vi "Kurven anzeigen.vi"() -> ()   [LabVIEW 2020, in "Grafik.lvlib"]
uses:
  Grafik.lvlib
  Visualisierungs Elemente/Button.ctl
  FT-IR/FGV FT-IR Gasliste Aktionen.ctl
  Messdaten/Aktionen FGV Messdaten.ctl
  Gaszuordnung AO/FGV Gaszuordnung Gas-Auswahl Aktion.ctl
  Messdaten/Messdaten.lvlib
  FT-IR/FT-IR.lvlib
  Gaszuordnung AO/Gaszuordnung AO.lvlib
  Allgemein/allgemeine Sub-VIs.lvlib
panel:
  in  "Clear":T1 caption="Beenden"
  in  "Beenden":T1
  in  "Komponenten":T2 {"Komponente 6" items=["---", "NO (3000) LP 191C", "NO2 (150) LP 191C (1of2)", "NO2 (2000) LP 191C (2of2)", "N2O (300) LP 191C (1of2)", "NH3 (300) LP 191C (1of2)", "NH3 (900,3000) LP 191C (2of2)", "HNCO (400) 191C", "H2O% (30) LP 191C", "Formaldehyde (70,500) LP 191C", "CO2 low% (4) LP 191C (2of2)", "CO2% (20) LP 191C (1of2)", "CO (700) LP 191C (1of3)", "CO% (1) LP 191C (2of3)", "Propylene (1000) LP 191C", "Aromatic HC C7 (500) LP 191C", "Ethylene (1000) LP 191C", "CH4 (250) LP 191C (1of2)", "CH4 (5000) LP 191C (2of2)", "Ethane (1000) LP 191C", "Acetylene (1000) LP 191C", "HNO2 (20) 191C", "MeOH (1000) 191C", "CO% (10) LP 191C (3of3)", "Formic Acid (100) 191C", "SO2 (500) LP 191C", "Acetaldehyde (1000) LP 191C", "COS (100) LP 191C", "1,3 butadiene (100) LP 191C", "Oil as Octane (200) LP 191C", "N2O (1000) LP 191C (2of2)", "Propane (200) LP 191C", "NO2 autorange (2000)", "CO autorange (100000)", "CH4 autorange (5000)", "NH3 autorange (3000)", "NOx autorange (3000)", "HCD (10000)", "NMHCD (10000)", "CO2% autorange (20)", "H2Oppm (300000)", "N2O autorange (1000)", "NMNEHCD (3000)", "Temp. Messzelle", "Druck Messzelle", "sBeam@2500", "Temp. HL zu FT-IR", "Temp. HL Extern SP1", "Austrittstemp. FT-IR", "Temp. Schaltschrank", "Konstant 0", "Konstant 50", "Konstant 100", "AK DUMMY"]; "Komponente 5" items=["---", "NO (3000) LP 191C", "NO2 (150) LP 191C (1of2)", "NO2 (2000) LP 191C (2of2)", "N2O (300) LP 191C (1of2)", "NH3 (300) LP 191C (1of2)", "NH3 (900,3000) LP 191C (2of2)", "HNCO (400) 191C", "H2O% (30) LP 191C", "Formaldehyde (70,500) LP 191C", "CO2 low% (4) LP 191C (2of2)", "CO2% (20) LP 191C (1of2)", "CO (700) LP 191C (1of3)", "CO% (1) LP 191C (2of3)", "Propylene (1000) LP 191C", "Aromatic HC C7 (500) LP 191C", "Ethylene (1000) LP 191C", "CH4 (250) LP 191C (1of2)", "CH4 (5000) LP 191C (2of2)", "Ethane (1000) LP 191C", "Acetylene (1000) LP 191C", "HNO2 (20) 191C", "MeOH (1000) 191C", "CO% (10) LP 191C (3of3)", "Formic Acid (100) 191C", "SO2 (500) LP 191C", "Acetaldehyde (1000) LP 191C", "COS (100) LP 191C", "1,3 butadiene (100) LP 191C", "Oil as Octane (200) LP 191C", "N2O (1000) LP 191C (2of2)", "Propane (200) LP 191C", "NO2 autorange (2000)", "CO autorange (100000)", "CH4 autorange (5000)", "NH3 autorange (3000)", "NOx autorange (3000)", "HCD (10000)", "NMHCD (10000)", "CO2% autorange (20)", "H2Oppm (300000)", "N2O autorange (1000)", "NMNEHCD (3000)", "Temp. Messzelle", "Druck Messzelle", "sBeam@2500", "Temp. HL zu FT-IR", "Temp. HL Extern SP1", "Austrittstemp. FT-IR", "Temp. Schaltschrank", "Konstant 0", "Konstant 50", "Konstant 100", "AK DUMMY"]; "Komponente 4" items=["---", "NO (3000) LP 191C", "NO2 (150) LP 191C (1of2)", "NO2 (2000) LP 191C (2of2)", "N2O (300) LP 191C (1of2)", "NH3 (300) LP 191C (1of2)", "NH3 (900,3000) LP 191C (2of2)", "HNCO (400) 191C", "H2O% (30) LP 191C", "Formaldehyde (70,500) LP 191C", "CO2 low% (4) LP 191C (2of2)", "CO2% (20) LP 191C (1of2)", "CO (700) LP 191C (1of3)", "CO% (1) LP 191C (2of3)", "Propylene (1000) LP 191C", "Aromatic HC C7 (500) LP 191C", "Ethylene (1000) LP 191C", "CH4 (250) LP 191C (1of2)", "CH4 (5000) LP 191C (2of2)", "Ethane (1000) LP 191C", "Acetylene (1000) LP 191C", "HNO2 (20) 191C", "MeOH (1000) 191C", "CO% (10) LP 191C (3of3)", "Formic Acid (100) 191C", "SO2 (500) LP 191C", "Acetaldehyde (1000) LP 191C", "COS (100) LP 191C", "1,3 butadiene (100) LP 191C", "Oil as Octane (200) LP 191C", "N2O (1000) LP 191C (2of2)", "Propane (200) LP 191C", "NO2 autorange (2000)", "CO autorange (100000)", "CH4 autorange (5000)", "NH3 autorange (3000)", "NOx autorange (3000)", "HCD (10000)", "NMHCD (10000)", "CO2% autorange (20)", "H2Oppm (300000)", "N2O autorange (1000)", "NMNEHCD (3000)", "Temp. Messzelle", "Druck Messzelle", "sBeam@2500", "Temp. HL zu FT-IR", "Temp. HL Extern SP1", "Austrittstemp. FT-IR", "Temp. Schaltschrank", "Konstant 0", "Konstant 50", "Konstant 100", "AK DUMMY"]; "Komponente 3" items=["---", "NO (3000) LP 191C", "NO2 (150) LP 191C (1of2)", "NO2 (2000) LP 191C (2of2)", "N2O (300) LP 191C (1of2)", "NH3 (300) LP 191C (1of2)", "NH3 (900,3000) LP 191C (2of2)", "HNCO (400) 191C", "H2O% (30) LP 191C", "Formaldehyde (70,500) LP 191C", "CO2 low% (4) LP 191C (2of2)", "CO2% (20) LP 191C (1of2)", "CO (700) LP 191C (1of3)", "CO% (1) LP 191C (2of3)", "Propylene (1000) LP 191C", "Aromatic HC C7 (500) LP 191C", "Ethylene (1000) LP 191C", "CH4 (250) LP 191C (1of2)", "CH4 (5000) LP 191C (2of2)", "Ethane (1000) LP 191C", "Acetylene (1000) LP 191C", "HNO2 (20) 191C", "MeOH (1000) 191C", "CO% (10) LP 191C (3of3)", "Formic Acid (100) 191C", "SO2 (500) LP 191C", "Acetaldehyde (1000) LP 191C", "COS (100) LP 191C", "1,3 butadiene (100) LP 191C", "Oil as Octane (200) LP 191C", "N2O (1000) LP 191C (2of2)", "Propane (200) LP 191C", "NO2 autorange (2000)", "CO autorange (100000)", "CH4 autorange (5000)", "NH3 autorange (3000)", "NOx autorange (3000)", "HCD (10000)", "NMHCD (10000)", "CO2% autorange (20)", "H2Oppm (300000)", "N2O autorange (1000)", "NMNEHCD (3000)", "Temp. Messzelle", "Druck Messzelle", "sBeam@2500", "Temp. HL zu FT-IR", "Temp. HL Extern SP1", "Austrittstemp. FT-IR", "Temp. Schaltschrank", "Konstant 0", "Konstant 50", "Konstant 100", "AK DUMMY"]; "Komponente 2" items=["---", "NO (3000) LP 191C", "NO2 (150) LP 191C (1of2)", "NO2 (2000) LP 191C (2of2)", "N2O (300) LP 191C (1of2)", "NH3 (300) LP 191C (1of2)", "NH3 (900,3000) LP 191C (2of2)", "HNCO (400) 191C", "H2O% (30) LP 191C", "Formaldehyde (70,500) LP 191C", "CO2 low% (4) LP 191C (2of2)", "CO2% (20) LP 191C (1of2)", "CO (700) LP 191C (1of3)", "CO% (1) LP 191C (2of3)", "Propylene (1000) LP 191C", "Aromatic HC C7 (500) LP 191C", "Ethylene (1000) LP 191C", "CH4 (250) LP 191C (1of2)", "CH4 (5000) LP 191C (2of2)", "Ethane (1000) LP 191C", "Acetylene (1000) LP 191C", "HNO2 (20) 191C", "MeOH (1000) 191C", "CO% (10) LP 191C (3of3)", "Formic Acid (100) 191C", "SO2 (500) LP 191C", "Acetaldehyde (1000) LP 191C", "COS (100) LP 191C", "1,3 butadiene (100) LP 191C", "Oil as Octane (200) LP 191C", "N2O (1000) LP 191C (2of2)", "Propane (200) LP 191C", "NO2 autorange (2000)", "CO autorange (100000)", "CH4 autorange (5000)", "NH3 autorange (3000)", "NOx autorange (3000)", "HCD (10000)", "NMHCD (10000)", "CO2% autorange (20)", "H2Oppm (300000)", "N2O autorange (1000)", "NMNEHCD (3000)", "Temp. Messzelle", "Druck Messzelle", "sBeam@2500", "Temp. HL zu FT-IR", "Temp. HL Extern SP1", "Austrittstemp. FT-IR", "Temp. Schaltschrank", "Konstant 0", "Konstant 50", "Konstant 100", "AK DUMMY"]; "Komponente 1" items=["---", "NO (3000) LP 191C", "NO2 (150) LP 191C (1of2)", "NO2 (2000) LP 191C (2of2)", "N2O (300) LP 191C (1of2)", "NH3 (300) LP 191C (1of2)", "NH3 (900,3000) LP 191C (2of2)", "HNCO (400) 191C", "H2O% (30) LP 191C", "Formaldehyde (70,500) LP 191C", "CO2 low% (4) LP 191C (2of2)", "CO2% (20) LP 191C (1of2)", "CO (700) LP 191C (1of3)", "CO% (1) LP 191C (2of3)", "Propylene (1000) LP 191C", "Aromatic HC C7 (500) LP 191C", "Ethylene (1000) LP 191C", "CH4 (250) LP 191C (1of2)", "CH4 (5000) LP 191C (2of2)", "Ethane (1000) LP 191C", "Acetylene (1000) LP 191C", "HNO2 (20) 191C", "MeOH (1000) 191C", "CO% (10) LP 191C (3of3)", "Formic Acid (100) 191C", "SO2 (500) LP 191C", "Acetaldehyde (1000) LP 191C", "COS (100) LP 191C", "1,3 butadiene (100) LP 191C", "Oil as Octane (200) LP 191C", "N2O (1000) LP 191C (2of2)", "Propane (200) LP 191C", "NO2 autorange (2000)", "CO autorange (100000)", "CH4 autorange (5000)", "NH3 autorange (3000)", "NOx autorange (3000)", "HCD (10000)", "NMHCD (10000)", "CO2% autorange (20)", "H2Oppm (300000)", "N2O autorange (1000)", "NMNEHCD (3000)", "Temp. Messzelle", "Druck Messzelle", "sBeam@2500", "Temp. HL zu FT-IR", "Temp. HL Extern SP1", "Austrittstemp. FT-IR", "Temp. Schaltschrank", "Konstant 0", "Konstant 50", "Konstant 100", "AK DUMMY"]}
  out "Grafik":cluster{"Zeitstempeln":timestamp[], dbl[]}[](graph)
  # "Grafik"
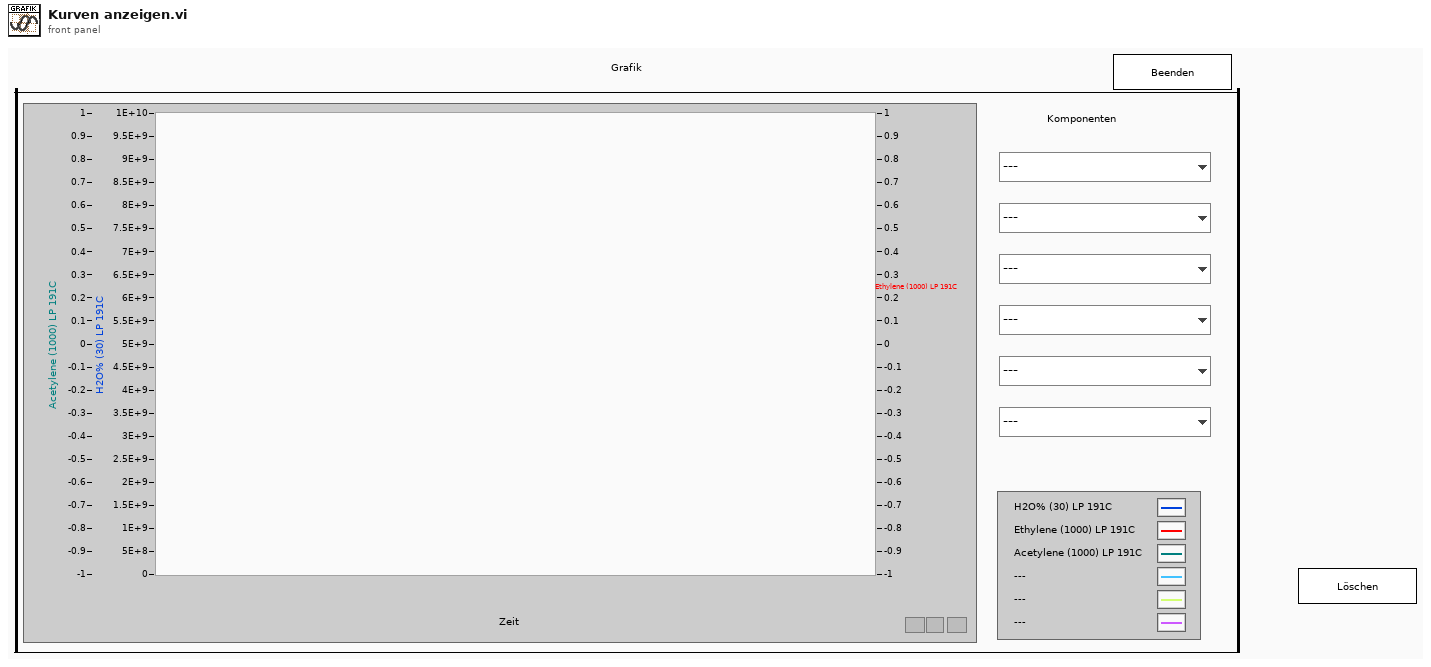
[diagram p1: front panel]
types:
  T1 = typedef "Button.ctl" = bool
  T2 = cluster{"Komponente 1":u16, "Komponente 2":u16, "Komponente 3":u16, "Komponente 4":u16, "Komponente 5":u16, "Komponente 6":u16}
  T3 = typedef "FT-IR.lvlib/FGV FT-IR Gasliste Aktionen.ctl" = enum16{"lesen", "Gasliste FT-IR", "Gasliste ausgelesen", "laden", "speichern", "löschen"}
  T4 = typedef "Gaszuordnung AO.lvlib/FGV Gaszuordnung Gas-Auswahl Aktion.ctl" = enum16{"Lesen", "AO Auswahl", "Graph Auswahl", "aktiver Graph", "laden", "speichern"}
  T5 = typedef "Messdaten.lvlib/Aktionen FGV Messdaten.ctl" = enum16{"lesen", "schreiben", "löschen", "Mittelwerte", "Komponente"}
  T6 = typedef "String - Ausgabefeld.ctl" = string
  T7 = typedef "Grafik.lvlib/Graphen Auswahl.ctl" = u16[]
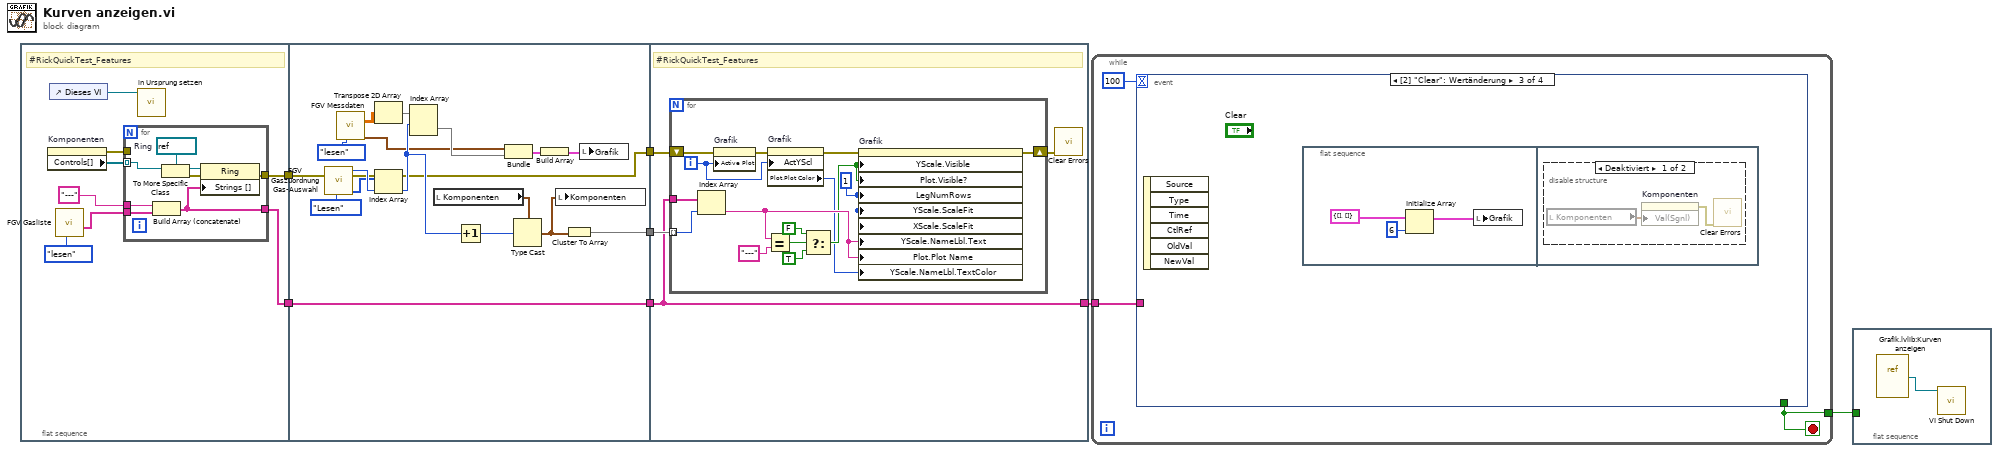
[diagram p0: block diagram]
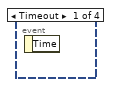
[diagram p2: hidden frame]
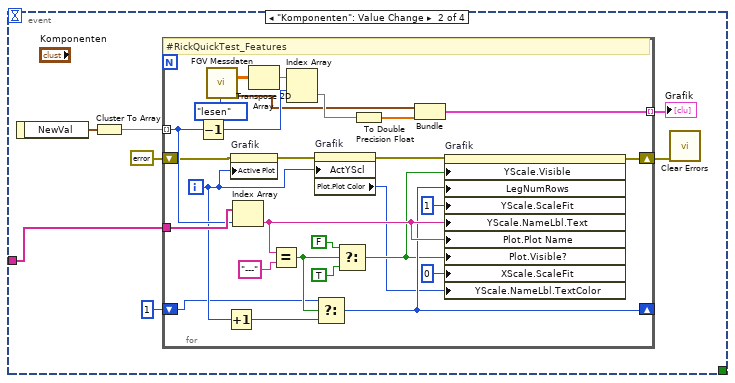
[diagram p3: hidden frame]
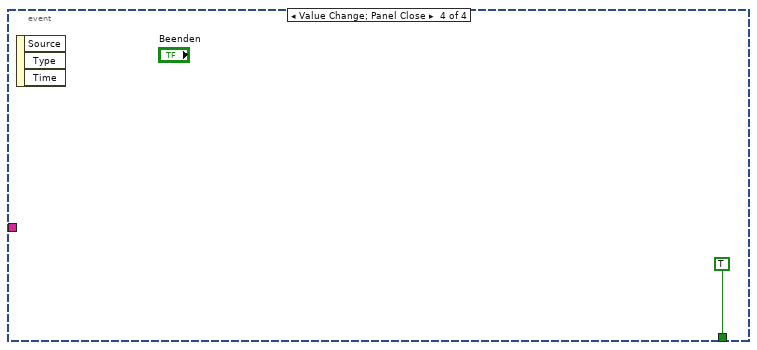
[diagram p5: hidden frame]
diagram:
  n1 = flat-sequence {
    tunnel: [w10] -> w7
    tunnel: [w9] -> w6
    tunnel: w7 -> [w24]
    tunnel: w6 -> [w31]
    tunnel: [w31] -> w5
    tunnel: [w29] -> w4
    tunnel: [w24] -> w1
    tunnel: w5 -> [w43]
    tunnel: w4 -> [w44]
    tunnel: [w43] -> w3
    tunnel: w1 -> [w42]
    frame #0 {
      # "#RickQuickTest_Features"
      n2 = property on="Komponenten" class="Cluster (strikt)"() -> (error out=w11:errorcluster, "Controls[]"=w12:refnum<vi>[])  [unwired: 2 in, 1 out]
      n3 = control-ref of="Dieses VI"() -> (w8:refnum<vi>)
      n4 = call "FGV Gasliste.vi"("Aktionen"=FGV_FT-IR_Gasliste_Aktionen."lesen") -> ("Aktuelle Gasliste gesamt"=w13:T6[])  [unwired: 8 in, 2 out]
      n5 = for {
        tunnel: "---" ("String") -> [w22]
        tunnel: w13 -> [w21]
        tunnel: w12 -> [w20] mode=indexing
        tunnel: w11 -> [_]
        tunnel: [w17] -> w10
        tunnel: [w16] -> w9
        w23 = refnum<vi> refnum  # Ring
        n6 = Build Array (concatenate)(w22, w21) -> (w16:T6[])
        n7 = To More Specific Class(target class=w23, reference=w20) -> (specific class reference=w19:refnum<vi>, error out=w18:errorcluster)  [unwired: 1 in]
        n8 = property class="Ring"(reference=w19, error in=w18, "Strings []"=w16) -> (error out=w17:errorcluster)  [unwired: 1 out]
      }
      n9 = call "in Ursprung setzen.vi"("VI Referenz"=w8) -> ()  [unwired: 10 in, 1 out]
    }
    frame #1 {
      n10 = call "FGV Gaszuordnung Gas-Auswahl.vi"("Aktion"=FGV_Gaszuordnung_Gas-Auswahl_Aktion."Lesen") -> ("Graphen"=w37:T7, "aktiver Graph"=w38:i32)  [unwired: 8 in, 1 out]
      n11 = call "FGV Messdaten.vi"("Aktionen"=Aktionen_FGV_Messdaten."lesen") -> ("Messdaten"=w35:sgl[][], "Zeitstempeln"=w25:timestamp[])  [unwired: 6 in, 7 out]
      n12 = Transpose 2D Array(2D array=w35) -> (transposed array=w34:sgl[][])
      n13 = Index Array(array=w37, index=w38) -> (element=w39:u16)
      n14 = Index Array(array=w34, index (row)=w39) -> (element=w28:sgl[])  [unwired: 1 in]
      n15 = local read "Komponenten"() -> (w40:T2)
      n16 = Increment(x=w39) -> (x+1=w32:u16)
      n17 = Bundle("Zeitstempeln"=w25, w28) -> (w27:cluster{"Zeitstempeln":timestamp[], sgl[]})  [unwired: 1 in]
      n18 = Type Cast(type=w40, x=w32) -> (*(type *) &x=w30:T2)
      n19 = Build Array(w27) -> (w26:cluster{"Zeitstempeln":timestamp[], sgl[]}[])
      n20 = local write "Komponenten"(w30) -> ()
      n21 = Cluster To Array(cluster=w30) -> (array=w29:u16[])
      n22 = local write "Grafik"(w26) -> ()
    }
    frame #2 {
      # "#RickQuickTest_Features"
      n23 = for {
        tunnel: w44 -> [w53] mode=indexing
        tunnel: w43 -> [w52]
        shift-right: [w50] -> w41
        shift-left: w42 -> [w45]
        i -> [w51]
        w48 = u8 1 ("Y-Achse.Achsenanpassung")
        n24 = Index Array(array=w52, index=w53) -> (element=w49:T6)
        n25 = property on="Grafik" class="XYGraph (strikt)"(error in=w45, "Active Plot"=w51) -> (error out=w54:errorcluster)  [unwired: 1 in, 1 out]
        n26 = Equal?(x=w49, y="---" ("String")) -> (x = y?=w58:bool)
        n27 = property on="Grafik" class="XYGraph (strikt)"(error in=w54, "ActYScl"=w51) -> (error out=w55:errorcluster, "Plot.Plot Color"=w46:u32)  [unwired: 1 in, 1 out]
        n28 = Select(t=FALSE, s=w58, f=TRUE) -> (s? t:f=w47:bool)
        n29 = property on="Grafik" class="XYGraph (strikt)"(error in=w55, "YScale.Visible"=w47, "Plot.Visible?"=w47, "LegNumRows"=w48, "YScale.ScaleFit"=w48, "XScale.ScaleFit"=w48, "YScale.NameLbl.Text"=w49, "Plot.Plot Name"=w49, "YScale.NameLbl.TextColor"=w46) -> (error out=w50:errorcluster)  [unwired: 1 in, 1 out]
      }
      n30 = call <vilib>:"Clear Errors.vi"("error in (no error)"=w41) -> ()  [unwired: 5 in, 2 out]
    }
  }
  n31 = while {
    tunnel: w3 -> [w61]
    tunnel: [w60] -> w2
    stop <- w60 stop-if-true
    n32 = event shown="[2] \"Clear\": Wertänderung" {
      selector: _ -> [_ _ _ _]
      dyn-events: _ -> [_ _ _ _]
      timeout: 100 -> [_ _ _ _]
      tunnel: [_ _ _ TRUE] -> w60
      tunnel: w61 -> [_ w67 _ _]
      event Timeout {
        n33 = event-data() -> ()  [unwired: 1 in, 1 out]
      }
      event "Komponenten": Value Change {
        n34 = event-data() -> ("NewVal"=w69:T2)  [unwired: 1 in]
        n35 = Cluster To Array(cluster=w69) -> (array=w68:u16[])
        n36 = for {
          tunnel: w68 -> [w80] mode=indexing
          tunnel: [w85] -> w66 mode=indexing
          tunnel: w67 -> [w89]
          shift-right: [w74] -> _
          shift-left: 1 -> [w76]
          shift-right: [w93] -> w63
          shift-left: errorcluster {"status"=FALSE, "code"=0, "source"=""} ("Fehler (Ausgang)") -> [w71]
          i -> [w77]
          # "#RickQuickTest_Features"
          n37 = Decrement(x=w80) -> (x-1=w88:u16)
          n38 = call "FGV Messdaten.vi"("Aktionen"=Aktionen_FGV_Messdaten."lesen") -> ("Messdaten"=w96:sgl[][], "Zeitstempeln"=w82:timestamp[])  [unwired: 6 in, 7 out]
          n39 = Increment(x=w77) -> (x+1=w75:i32)
          n40 = property on="Grafik" class="XYGraph (strikt)"(error in=w71, "Active Plot"=w77) -> (error out=w92:errorcluster)  [unwired: 1 in, 1 out]
          n41 = Index Array(array=w89, index=w80) -> (element=w81:T6)
          n42 = Transpose 2D Array(2D array=w96) -> (transposed array=w95:sgl[][])
          n43 = Equal?(x=w81, y="---" ("String")) -> (x = y?=w78:bool)
          n44 = Index Array(array=w95, index (row)=w88) -> (element=w84:sgl[])  [unwired: 1 in]
          n45 = property on="Grafik" class="XYGraph (strikt)"(error in=w92, "ActYScl"=w77) -> (error out=w91:errorcluster, "Plot.Plot Color"=w70:u32)  [unwired: 1 in, 1 out]
          n46 = Select(t=w76, s=w78, f=w75) -> (s? t:f=w74:i32)
          n47 = Select(t=FALSE, s=w78, f=TRUE) -> (s? t:f=w73:bool)
          n48 = To Double Precision Float(number=w84) -> (double precision float=w83:dbl[])
          n49 = Bundle("Zeitstempeln"=w82, w83) -> (w85:cluster{"Zeitstempeln":timestamp[], dbl[]})  [unwired: 1 in]
          n50 = property on="Grafik" class="XYGraph (strikt)"(error in=w91, "YScale.Visible"=w73, "LegNumRows"=w74, "YScale.ScaleFit"=u8 1 ("Y-Achse.Achsenanpassung"), "YScale.NameLbl.Text"=w81, "Plot.Plot Name"=w81, "Plot.Visible?"=w73, "XScale.ScaleFit"=u8 0 ("X-Achse.Achsenanpassung"), "YScale.NameLbl.TextColor"=w70) -> (error out=w93:errorcluster)  [unwired: 1 in, 1 out]
        }
        "Grafik" <- w66
        n51 = call <vilib>:"Clear Errors.vi"("error in (no error)"=w63) -> ()  [unwired: 5 in, 2 out]
      }
      event Value Change {
        n52 = event-data() -> ()  [unwired: 1 in, 6 out]
        n53 = flat-sequence {
          frame #0 {
            n54 = Initialize Array(cluster{"Zeitstempeln":timestamp[], dbl[]} {"Zeitstempeln"=[], []}, 6 ("Dimensionsgröße")) -> (w98:cluster{"Zeitstempeln":timestamp[], dbl[]}[])
            n55 = local write "Grafik"(w98) -> ()
          }
          frame #1 {
            n56 = disable-structure shown="Deaktiviert" {
              frame Disabled {
                n57 = local read "Komponenten"() -> (w101:T2)
                n58 = property on="Komponenten" class="Cluster (strikt)"("Val(Sgnl)"=w101) -> (error out=w100:errorcluster)  [unwired: 2 in, 1 out]
                n59 = call <vilib>:"Clear Errors.vi"("error in (no error)"=w100) -> ()  [unwired: 5 in, 2 out]
              }
              frame Enabled {
              }
            }
          }
        }
      }
      event Value Change; Panel Close {
        n60 = event-data() -> ()  [unwired: 1 in, 3 out]
      }
    }
  }
  n61 = flat-sequence {
    tunnel: w2 -> [_]
    frame #0 {
      n62 = vi-ref "Grafik.lvlib:Kurven anzeigen.vi"() -> (w103:refnum<vi>)
      n63 = call "VI Shut Down.vi"("VI Referenz"=w103) -> ()  [unwired: 11 in]
    }
  }
